vi "BETA - 0.1 - Motor Slower - David G.vi"(6 "%":dbl min=0.0 max=25.0, 8 "Backward Limit":dbl, 9 "Forward Limit":dbl, 10 "Speed":dbl min=0.0 max=25.0, 11 "Encoder Value":dbl) -> (2 "Speed Output":dbl)   [LabVIEW 2018]
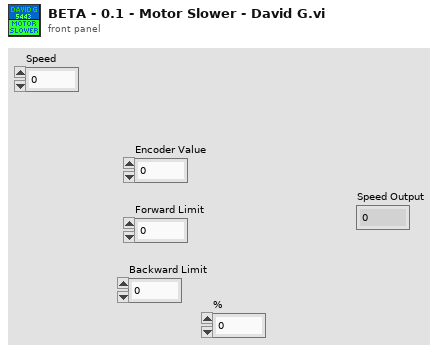
[diagram p1: front panel]
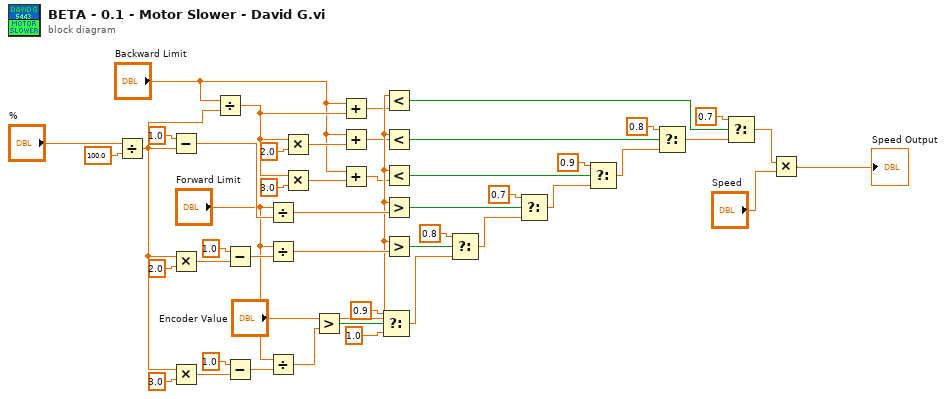
[diagram p0: block diagram]
diagram:
  n1 = Divide(x="%", y=100.0) -> (x/y=w24:dbl)
  n2 = Subtract(x=1.0, y=w24) -> (x-y=w44:dbl)
  n3 = Multiply(x=w24, y=2.0) -> (x*y=w31:dbl)
  n4 = Multiply(x=w24, y=3.0) -> (x*y=w27:dbl)
  n5 = Divide(x="Backward Limit", y=w24) -> (x/y=w7:dbl)
  n6 = Subtract(x=1.0, y=w31) -> (x-y=w33:dbl)
  n7 = Subtract(x=1.0, y=w27) -> (x-y=w26:dbl)
  n8 = Divide(x="Forward Limit", y=w44) -> (x/y=w48:dbl)
  n9 = Divide(x="Forward Limit", y=w33) -> (x/y=w30:dbl)
  n10 = Divide(x="Forward Limit", y=w26) -> (x/y=w23:dbl)
  n11 = Multiply(x=w7, y=2.0) -> (x*y=w2:dbl)
  n12 = Multiply(x=w7, y=3.0) -> (x*y=w3:dbl)
  n13 = Greater?(x="Encoder Value", y=w23) -> (0:w35:bool)
  n14 = Add(x="Backward Limit", y=w7) -> (x+y=w6:dbl)
  n15 = Add(x="Backward Limit", y=w2) -> (x+y=w5:dbl)
  n16 = Add(x="Backward Limit", y=w3) -> (x+y=w4:dbl)
  n17 = Select(t=0.9, s=w35, f=1.0) -> (s? t:f=w40:dbl)
  n18 = Less?(x="Encoder Value", y=w6) -> (x < y?=w19:bool)
  n19 = Less?(x="Encoder Value", y=w5) -> (x < y?=w18:bool)
  n20 = Less?(x="Encoder Value", y=w4) -> (x < y?=w17:bool)
  n21 = Greater?(x="Encoder Value", y=w48) -> (0:w37:bool)
  n22 = Greater?(x="Encoder Value", y=w30) -> (0:w36:bool)
  n23 = Select(t=0.8, s=w36, f=w40) -> (s? t:f=w39:dbl)
  n24 = Select(t=0.7, s=w37, f=w39) -> (s? t:f=w13:dbl)
  n25 = Select(t=0.9, s=w17, f=w13) -> (s? t:f=w12:dbl)
  n26 = Select(t=0.8, s=w18, f=w12) -> (s? t:f=w11:dbl)
  n27 = Select(t=0.7, s=w19, f=w11) -> (s? t:f=w9:dbl)
  n28 = Multiply(x=w9, y="Speed") -> (x*y=→"Speed Output":dbl)
